vi "Parse Core(override).vi"(8 "error in (no error)":errorcluster, 11 "NI Generic Parser in":refnum<class "NI Generic Parser.lvclass">) -> (0 "error out":errorcluster, 2 "Measurements Out":T1[](array[typedef]), 3 "NI Generic Parser out":refnum<class "NI Generic Parser.lvclass">)   [LabVIEW 2016, in "NI Generic Parser.lvlib" / "NI Generic Parser.lvclass"]
uses:
  NI Generic Parser.lvclass
  Plugins/File Parsing Interface.lvlibp/Controls/Parsed Measurement.ctl
  Plugins/Measurement Data.lvlibp/Measurement Data.lvclass
  Plugins/File Parsing Interface.lvlibp/File Parsing Interface.lvclass
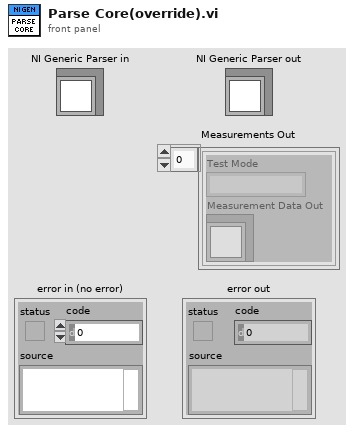
[diagram p1: front panel]
types:
  T1 = typedef "File Parsing Interface.lvlibp/File Parsing Interface.lvclass/Parsed Measurement.ctl" = cluster{"Test Mode":string, "Measurement Data Out":refnum<class "Measurement Data.lvclass">}
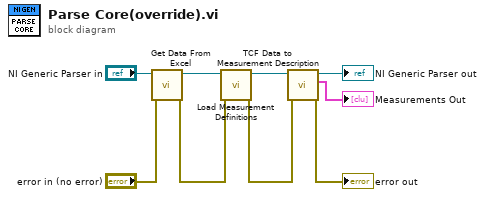
[diagram p0: block diagram]
diagram:
  n1 = call "Get Data From Excel.vi"("error in (no error)"="error in (no error)", "NI Generic Parser in"="NI Generic Parser in") -> ("error out"=w8:errorcluster, "NI Generic Parser out"=w5:refnum<class "NI Generic Parser.lvclass">)  [unwired: 8 in]
  n2 = call "Load Measurement Definitions.vi"("error in (no error)"=w8, "NI Generic Parser in"=w5) -> ("error out"=w6:errorcluster, "NI Generic Parser out"=w3:refnum<class "NI Generic Parser.lvclass">)  [unwired: 8 in]
  n3 = call "TCF Data to  Measurement Description.vi"("error in (no error)"=w6, "NI Generic Parser in"=w3) -> ("error out"=→"error out":errorcluster, "Measurements Out"=→"Measurements Out":T1[], "NI Generic Parser out"=→"NI Generic Parser out":refnum<class "NI Generic Parser.lvclass">)  [unwired: 7 in]
